vi "DAC_manual_set.vi"() -> ()   [LabVIEW 2013]
uses:
  <vilib>/FPGAPlugInAG/sbRIO-9602/niLvFpga_Close_sbRIO-9602.vi
  <vilib>/rvi/interface/nirviCloseFPGA/nirviCloseFPGA.xnode
  fpga-bitfile-ref.ctl
  FPGA Bitfiles/fpga-clean1_FPGATarget_FPGAMAINlock-in_FC21E42C.lvbitx
panel:
  in  "DAC param":T1={"IP Adress FPGA"="192.168.137.21", "Delay(ms)"=1, "Busses to use"=[TRUE, TRUE, TRUE, FALSE, FALSE, FALSE, FALSE, FALSE], "max"=0.3, "min"=-2.0}
  in  "Read":bool
  in  "Set":bool
  in  "Ramp":bool
  in  "All to":bool
  in  "All to":dbl
  in  "stop":bool
  in  "DAC control":dbl[][](array[numeric])=[[0.0, 0.0, 0.0, 0.0, 0.0, 0.0, 0.0, 0.0], [0.0, 0.0, 0.0, 0.0, 0.0, 0.0, 0.0, 0.0], [0.0, 0.0, 0.0, 0.0, 0.0, 0.0, 0.0, 0.0], [0.0, 0.0, 0.0, 0.0, 0.0, 0.0, 0.0, 0.0], [0.0, 0.0, 0.0, 0.0, 0.0, 0.0, 0.0, 0.0], [0.0, 0.0, 0.0, 0.0, 0.0, 0.0, 0.0, 0.0], [0.0, 0.0, 0.0, 0.0, 0.0, 0.0, 0.0, 0.0], [0.0, 0.0, 0.0, 0.0, 0.0, 0.0, 0.0, 0.0]]
  # "All to"
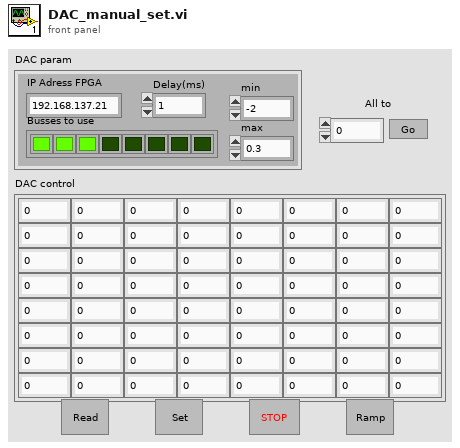
[diagram p1: front panel]
types:
  T1 = cluster{"IP Adress FPGA":string, "Delay(ms)":u8, "Busses to use":bool[], "max":dbl, "min":dbl}
  T2 = enum8{"start movement", "buses to use", "delay", "value", "stop", ""}
  T3 = enum8{"start movement", "buses to use", "delay", "value"}
  T4 = typedef "fpga-bitfile-ref.ctl" = refnum<k20>
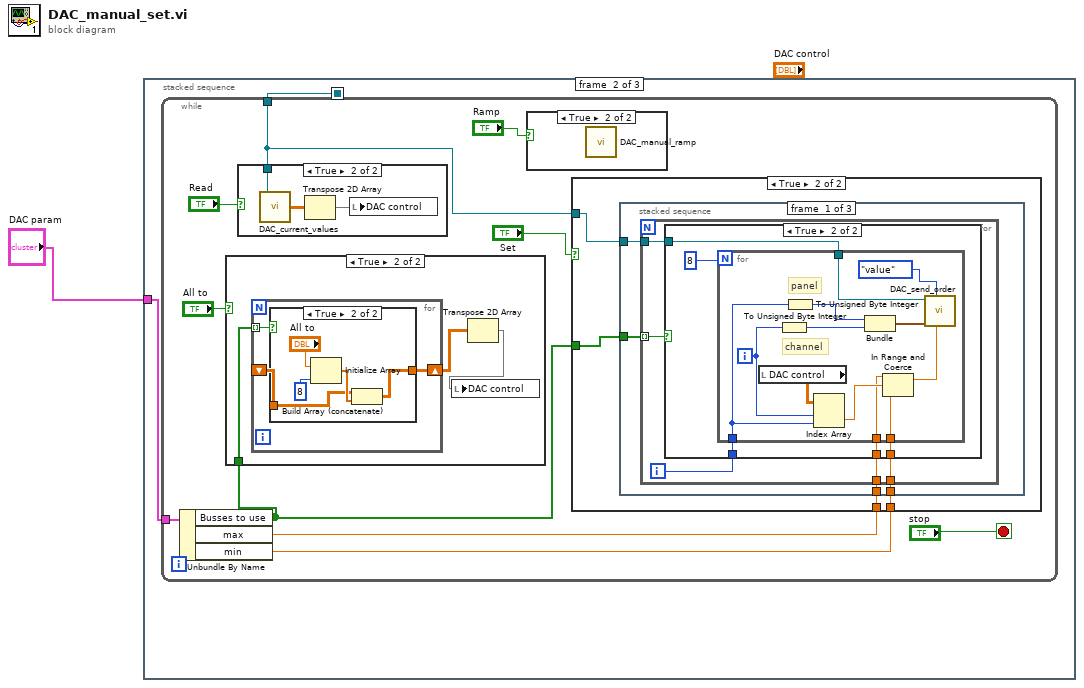
[diagram p0: block diagram]
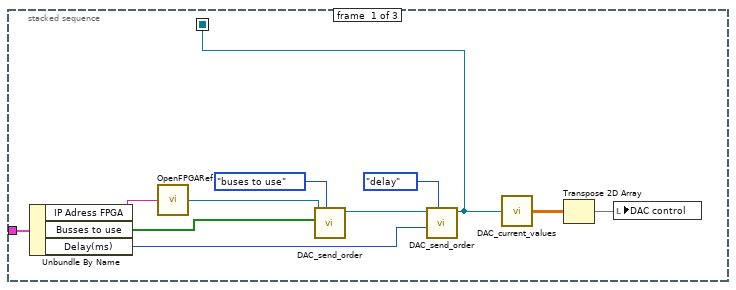
[diagram p2: hidden frame]
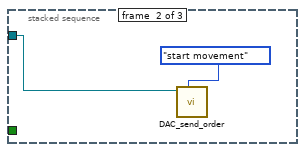
[diagram p6: hidden frame]
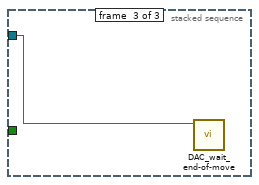
[diagram p7: hidden frame]
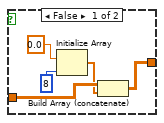
[diagram p9: hidden frame]
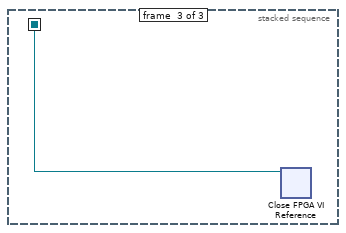
[diagram p11: hidden frame]
diagram:
  n1 = stacked-sequence {
    seq-local: [w8 _ _] -> [_ w14 w77]
    tunnel: "DAC param" -> [w4 w13 _]
    frame #0 {
      n2 = Unbundle By Name(w4) -> ("IP Adress FPGA"=w5:string, "Busses to use"=w3:bool[], "Delay(ms)"=w2:u8)
      n3 = call "OpenFPGARef.vi"("IP Address"=w5) -> ("FPGA VI Reference Out"=w9:T4)
      n4 = call "DAC_send_order.vi"("order"=T2."buses to use", "buses to use"=w3, "FPGA VI Reference In"=w9) -> ("FPGA VI Reference Out"=w10:T4)  [unwired: 8 in]
      n5 = call "DAC_send_order.vi"("order"=T2."delay", "delay between steps (ms)"=w2, "FPGA VI Reference In"=w10) -> ("FPGA VI Reference Out"=w8:T4)  [unwired: 8 in]
      n6 = call "DAC_current_values.vi"("FPGA Ref"=w8) -> ("DAC values"=w7:sgl[][])
      n7 = Transpose 2D Array(2D array=w7) -> (transposed array=w6:sgl[][])
      n8 = local write "DAC control"(w6) -> ()
    }
    frame #1 {
      n9 = while {
        tunnel: w14 -> [w16]
        tunnel: w13 -> [w20]
        stop <- "stop" stop-if-true
        n10 = Unbundle By Name(w20) -> ("Busses to use"=w19:bool[], "max"=w18:dbl, "min"=w17:dbl)
        n11 = case shown="True" "All to" {
          tunnel: w19 -> [_ w58]
          frame False {
          }
          frame True {
            n12 = for {
              shift-right: [w63] -> w60
              shift-left: _ -> [w62]
              tunnel: w58 -> [w61] mode=indexing
              n13 = case shown="True" w61 {
                tunnel: [w66 w71] -> w63
                tunnel: w62 -> [w67 w69]
                frame False {
                  n14 = Initialize Array(0.0, 8) -> (w65:dbl[])
                  n15 = Build Array (concatenate)(w67, w65) -> (w66:dbl[][])
                }
                frame True {
                  n16 = Initialize Array("All to", 8) -> (w72:dbl[])
                  n17 = Build Array (concatenate)(w69, w72) -> (w71:dbl[][])
                }
              }
            }
            n18 = Transpose 2D Array(2D array=w60) -> (transposed array=w59:dbl[][])
            n19 = local write "DAC control"(w59) -> ()
          }
        }
        n20 = case shown="True" "Read" {
          tunnel: w16 -> [_ w76]
          frame False {
          }
          frame True {
            n21 = call "DAC_current_values.vi"("FPGA Ref"=w76) -> ("DAC values"=w74:sgl[][])
            n22 = Transpose 2D Array(2D array=w74) -> (transposed array=w75:sgl[][])
            n23 = local write "DAC control"(w75) -> ()
          }
        }
        n24 = case shown="True" "Ramp" {
          frame False {
          }
          frame True {
            n25 = call "DAC_manual_ramp.vi"() -> ()  [unwired: 4 in]
          }
        }
        n26 = case shown="True" "Set" {
          tunnel: w16 -> [_ w28]
          tunnel: w19 -> [_ w27]
          tunnel: w18 -> [_ w26]
          tunnel: w17 -> [_ w25]
          frame False {
          }
          frame True {
            n27 = stacked-sequence {
              tunnel: w28 -> [w32 w55 w57]
              tunnel: w27 -> [w31 _ _]
              tunnel: w26 -> [w30 _ _]
              tunnel: w25 -> [w29 _ _]
              frame #0 {
                n28 = for {
                  tunnel: w32 -> [w37]
                  tunnel: w31 -> [w35] mode=indexing
                  tunnel: w30 -> [w34]
                  tunnel: w29 -> [w33]
                  i -> [w36]
                  n29 = case shown="True" w35 {
                    tunnel: w37 -> [_ w42]
                    tunnel: w36 -> [_ w40]
                    tunnel: w34 -> [_ w39]
                    tunnel: w33 -> [_ w38]
                    frame False {
                    }
                    frame True {
                      n30 = for {
                        N: 8 -> [_]
                        tunnel: w42 -> [w49]
                        tunnel: w40 -> [w46]
                        tunnel: w39 -> [w44]
                        tunnel: w38 -> [w43]
                        i -> [w47]
                        # "channel"
                        # "panel"
                        n31 = local read "DAC control"() -> (w48:dbl[][])
                        n32 = To Unsigned Byte Integer(number=w47) -> (unsigned 8bit integer=w52:u8)
                        n33 = To Unsigned Byte Integer(number=w46) -> (unsigned 8bit integer=w53:u8)
                        n34 = Index Array(array=w48, index (row)=w47, index (col)=w46) -> (element=w45:dbl)
                        n35 = Bundle(w53, w52) -> (w51:cluster{u8, u8})  [unwired: 1 in]
                        n36 = In Range and Coerce(upper limit=w44, x=w45, lower limit=w43) -> (coerced(x)=w50:dbl)  [unwired: 1 out]
                        n37 = call "DAC_send_order.vi"("DAC goto value"=w50, "order"=T3."value", "Cluster"=w51, "FPGA VI Reference In"=w49) -> ()  [unwired: 3 in, 5 out]
                      }
                    }
                  }
                }
              }
              frame #1 {
                n38 = call "DAC_send_order.vi"("order"=T3."start movement", "FPGA VI Reference In"=w55) -> ()  [unwired: 5 in, 5 out]
              }
              frame #2 {
                n39 = call "DAC_wait_end-of-move.vi"("FPGA VI Reference In"=w57) -> ()  [unwired: 10 in, 1 out]
              }
            }
          }
        }
      }
    }
    frame #2 {
      n40 = xnode "Close FPGA VI Reference"("FPGA VI Reference In"=w77) -> ()  [unwired: 1 in, 1 out]
    }
  }
